vi "Write Data.vi"(8 "error in":errorcluster, 10 "Data":waveform(dbl), 11 "Waveform Data in":refnum<class "Waveform Data.lvclass">) -> (0 "error out":errorcluster, 3 "Waveform Data out":refnum<class "Waveform Data.lvclass">)   [LabVIEW 2018, in "Base Data Class.lvlib" / "Waveform Data.lvclass"]
uses:
  Waveform Data.lvclass
  Waveform Data.lvclass/Waveform Data.ctl
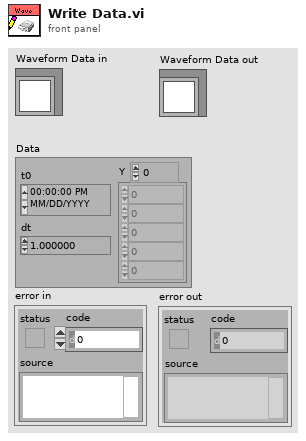
[diagram p1: front panel]
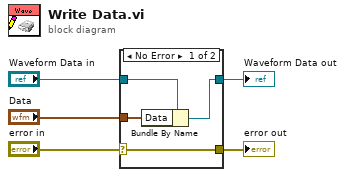
[diagram p0: block diagram]
diagram:
  n1 = case shown="No Error" "error in" {
    selector: "error in" -> [w9 w10]
    tunnel: [w9 w10] -> w4
    tunnel: [w7 w11] -> w2
    tunnel: "Waveform Data in" -> [w8 w11]
    tunnel: "Data" -> [w6 _]
    frame No Error {
      n2 = Bundle By Name(cluster=w8, "Data"=w6) -> (w7:refnum<class "Waveform Data.lvclass">)
    }
    frame Error {
    }
  }
  "error out" <- w4
  "Waveform Data out" <- w2
